vi "HumanExecuteCompitition.vi"(8 "error in (no error)":errorcluster) -> (0 "error out":errorcluster)   [LabVIEW 2023]
doc: "Execute for Human\n\ninput:\n error in (cluster)\n\noutput:\n error out (cluster)"
uses:
  <vilib>/Rock Robotics/WPI/Joystick/XBox Buttons Indexer.ctl
  <vilib>/Rock Robotics/WPI/Joystick/XBox Axes Indexer.ctl
  <vilib>/Rock Robotics/WPI/ThirdParty/JAS_Junk/TrajLib/VI/BoolCmd_Send_Internal.vi
  <vilib>/Rock Robotics/WPI/ThirdParty/JAS_Junk/TrajLib/VI/BoolCmd_ObtainQueue.vi
  HumanGlobal.vi
  <vilib>/Rock Robotics/Network Tables/NT Write String.vi
  <vilib>/Rock Robotics/WPI/ThirdParty/JAS_Junk/TrajLib/Trajectory_Library.lvlib
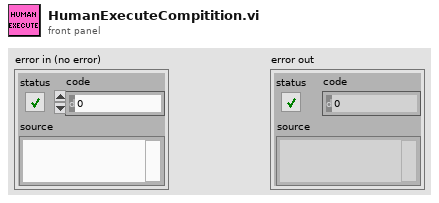
[diagram p1: front panel]
types:
  T1 = typedef "XBox Axes Indexer.ctl" = enum16{"Left X", "Left Y", "Left Trigger", "Right Trigger", "Right X", "Right Y"}
  T2 = typedef "XBox Buttons Indexer.ctl" = enum16{"A", "B", "X", "Y", "Left Bumper", "Right Bumper", "Back", "Start", "Left Joystick", "Right Joystick"}
  T3 = typedef "WPI_JoystickDevRef.ctl" = cluster{"Device":T4}
  T4 = typedef "WPI_JoystickDeviceEnum.ctl" = enum16{"USB 0", "USB 1", "USB 2", "USB 3", "USB 4", "USB 5"}
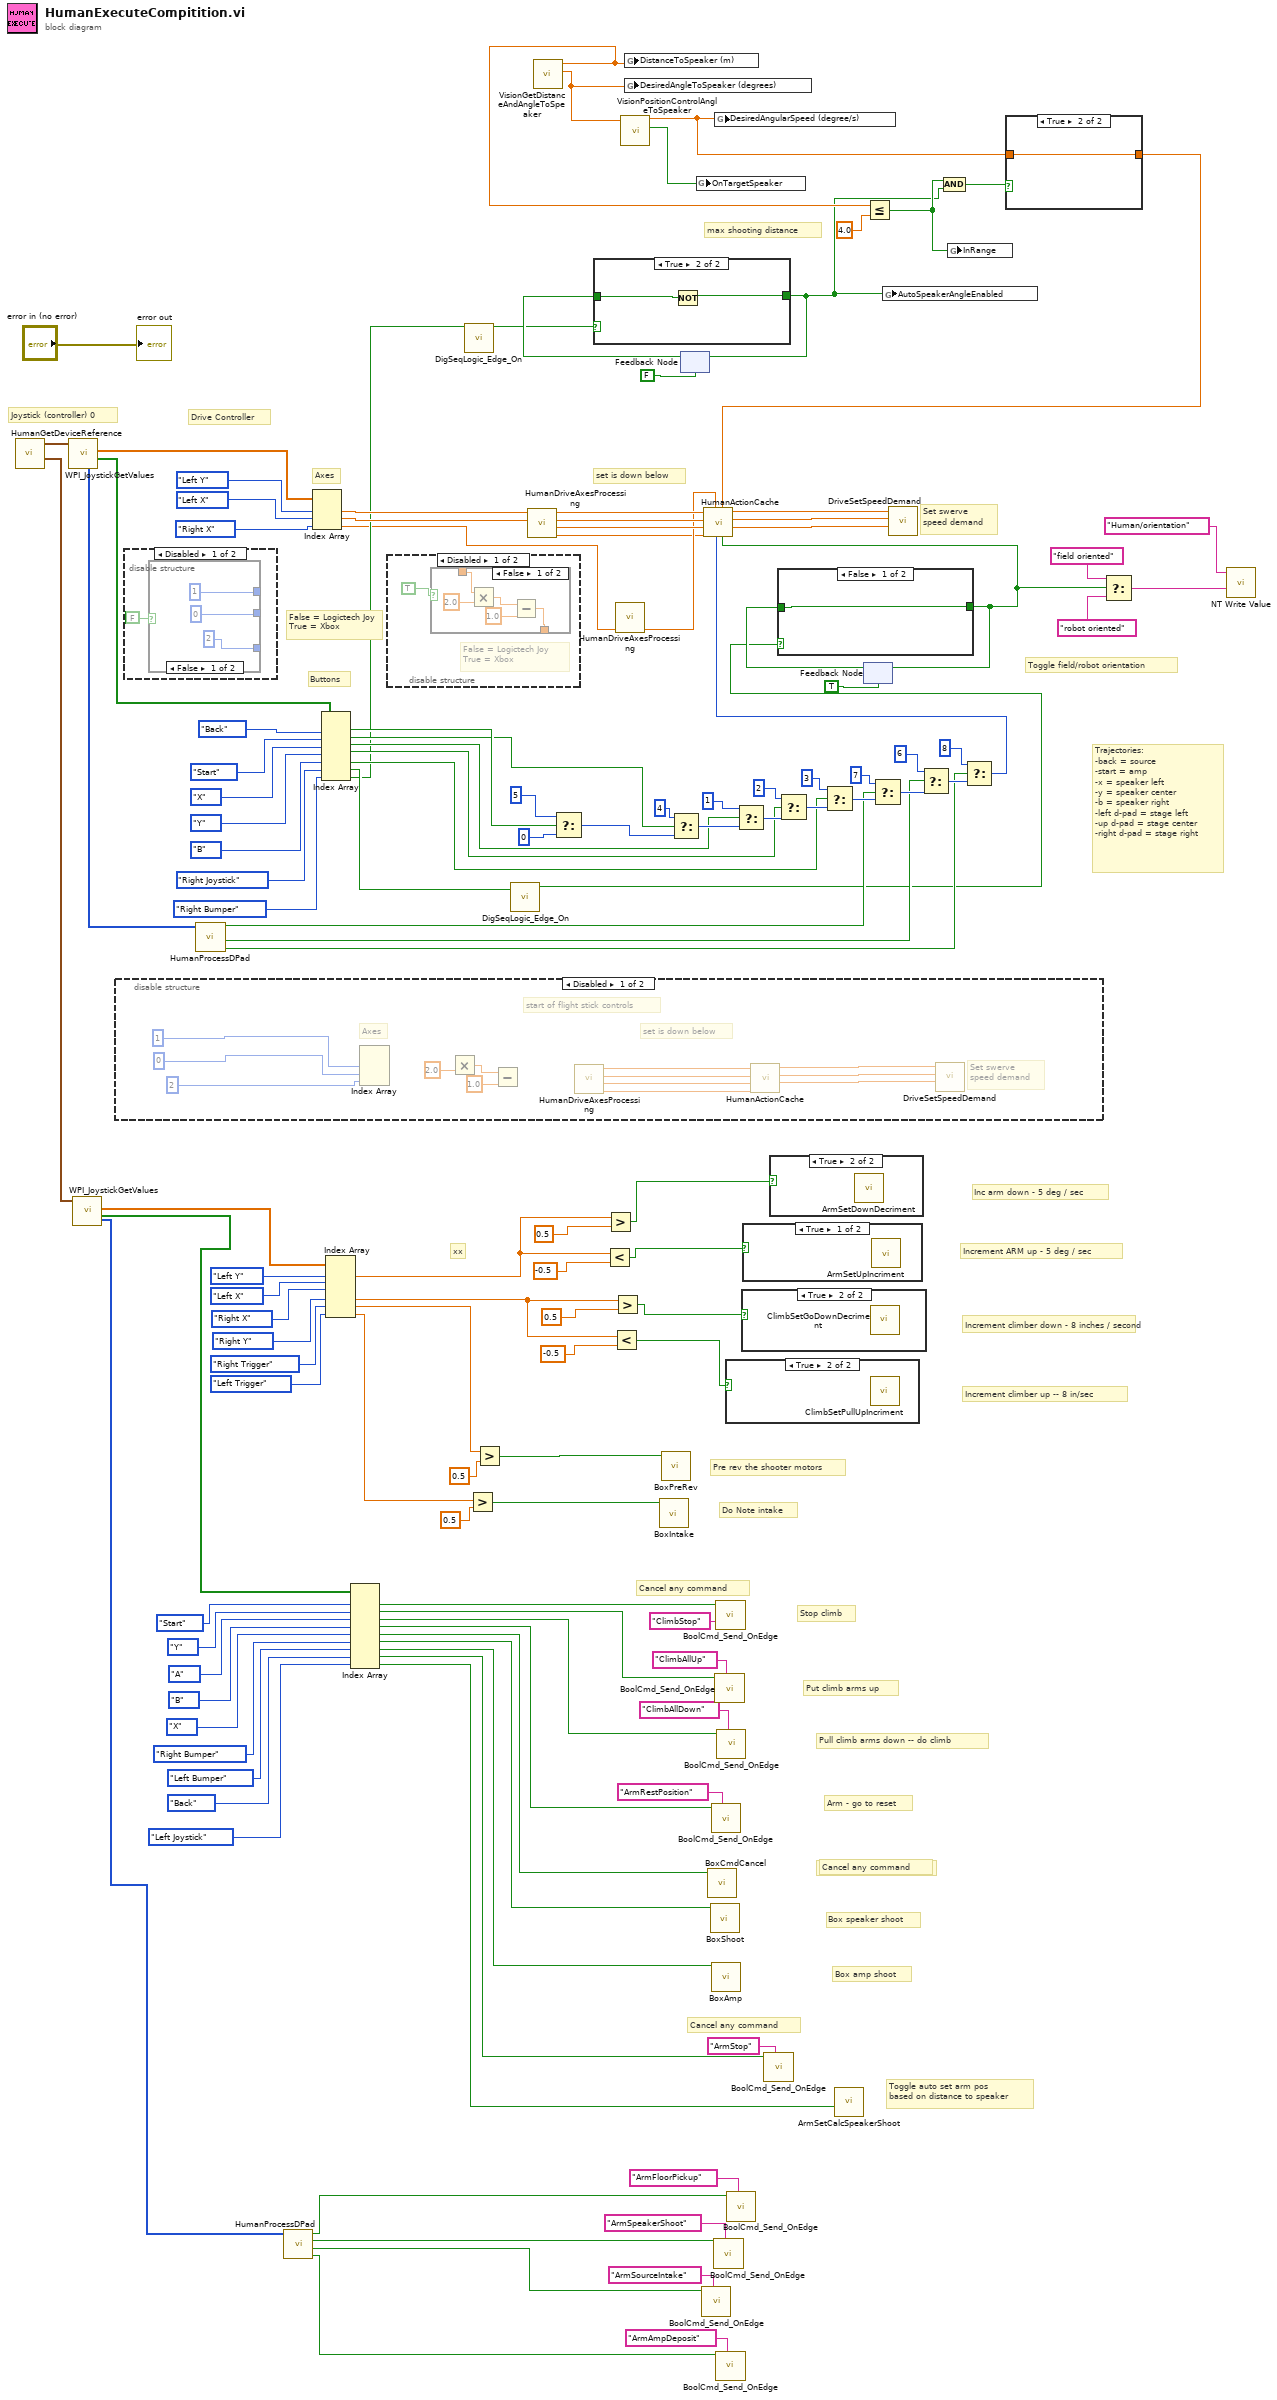
[diagram p0: block diagram]
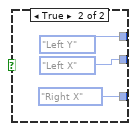
[diagram p3: hidden frame]
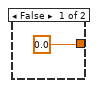
[diagram p8: hidden frame]
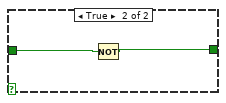
[diagram p9: hidden frame]
diagram:
  # "False = Logictech Joy\nTrue = Xbox"
  # "Toggle auto set arm pos\nbased on distance to speaker"
  # "Box amp shoot"
  # "Box speaker shoot"
  # "Box - cancel any action"
  # "Arm - go to reset"
  # "Pull climb arms down -- do climb"
  # "Put climb arms up"
  # "Stop climb"
  # "Increment ARM up - 5 deg / sec"
  # "Increment climber up -- 8 in/sec"
  # "Do Note intake"
  # "Pre rev the shooter motors"
  # "max shooting distance"
  # "Toggle field/robot orientation"
  # "Increment climber down - 8 inches / second"
  # "xx"
  # "Cancel any command"
  # "Cancel any command"
  # "Inc arm down - 5 deg / sec"
  # "Trajectories:\n-back = source\n-start = amp\n-x = speaker left\n-y = speaker center\n-b = speaker right\n-left d-pad = stage left\n-up d-pad = stage center\n-right d-pad = stage right"
  # "Buttons"
  # "Axes"
  # "Cancel any command"
  # "set is down below"
  # "Set swerve\nspeed demand"
  # "Joystick (controller) 0"
  # "Drive Controller"
  n1 = call "HumanGetDeviceReference.vi"() -> ("Aux Joy"=w116:T3, "Driver Joy"=w120:T3)  [unwired: 9 in, 1 out]
  n2 = call <vilib>:"WPI_JoystickGetValues.vi"("JoystickDevRef"=w120) -> ("Buttons"=w93:bool[], "Axes"=w102:dbl[], "POVs"=w129:i16[])  [unwired: 6 in, 2 out]
  n3 = call <vilib>:"WPI_JoystickGetValues.vi"("JoystickDevRef"=w116) -> ("Buttons"=w106:bool[], "Axes"=w115:dbl[], "POVs"=w68:i16[])  [unwired: 6 in, 2 out]
  n4 = disable-structure shown="Disabled" {
    frame Disabled {
      # "start of flight stick controls"
      # "Axes"
      # "set is down below"
      # "Set swerve\nspeed demand"
      n5 = Index Array(index #1=1, index #2=0, index #3=2) -> ()  [unwired: 1 in, 3 out]
      n6 = Multiply(y=2.0) -> (x*y=w132:dbl)  [unwired: 1 in]
      n7 = Subtract(x=w132, y=1.0) -> ()  [unwired: 1 out]
      n8 = call "HumanDriveAxesProcessing.vi"() -> ("Right X"=w137:dbl, "Right Y"=w142:dbl, "Left X"=w143:dbl, "Left Y"=w141:dbl)  [unwired: 8 in]
      n9 = call "HumanActionCache.vi"("Right X"=w137, "Right Y"=w142, "Left X"=w143, "Left Y"=w141) -> ("AMotorDemand"=w140:dbl, "YMotorDemand"=w139:dbl, "XMotorDemand"=w138:dbl)  [unwired: 5 in]
      n10 = call "DriveSetSpeedDemand.vi"("ASpeedDemand (d/s)"=w140, "YSpeedDemand (ft/s)"=w139, "XSpeedDemand (ft/s)"=w138) -> ()  [unwired: 9 in]
    }
    frame Enabled {
    }
  }
  n11 = disable-structure shown="Disabled" {
    frame Disabled {
      n12 = case shown="False" FALSE {
        tunnel: [1 XBox_Axes_Indexer."Left Y" ("XBox Axes")] -> _
        tunnel: [0 XBox_Axes_Indexer."Left X" ("XBox Axes")] -> _
        tunnel: [2 XBox_Axes_Indexer."Right X" ("XBox Axes")] -> _
        frame False {
        }
        frame True {
        }
      }
    }
    frame Enabled {
    }
  }
  n13 = call "HumanProcessDPad.vi"("POV"=w129) -> ("Right"=w46:bool, "Left"=w47:bool, "Up"=w48:bool)  [unwired: 7 in, 1 out]
  n14 = call "HumanProcessDPad.vi"("POV"=w68) -> ("Right"=w65:bool, "Left"=w63:bool, "Down"=w64:bool, "Up"=w66:bool)  [unwired: 7 in]
  n15 = Index Array(array=w102, index #1=XBox_Axes_Indexer."Left Y" ("XBox Axes"), index #2=XBox_Axes_Indexer."Left X" ("XBox Axes"), index #3=XBox_Axes_Indexer."Right X" ("XBox Axes")) -> (element #1=w128:dbl, element #2=w127:dbl, element #3=w5:dbl)
  n16 = Index Array(array=w93, index #1=XBox_Buttons_Indexer."Back" ("Nothing"), index #2=XBox_Buttons_Indexer."Start" ("Nothing"), index #3=XBox_Buttons_Indexer."X" ("Nothing"), index #4=XBox_Buttons_Indexer."Y" ("Nothing"), index #5=XBox_Buttons_Indexer."B" ("Nothing"), index #6=XBox_Buttons_Indexer."Right Joystick" ("Nothing"), index #7=XBox_Buttons_Indexer."Right Bumper" ("Nothing")) -> (element #1=w62:bool, element #2=w52:bool, element #3=w51:bool, element #4=w50:bool, element #5=w49:bool, element #6=w32:bool, element #7=w12:bool)
  n17 = Index Array(array=w115, index #1=XBox_Axes_Indexer."Left Y" ("XBox Axes"), index #2=XBox_Axes_Indexer."Left X" ("XBox Axes"), index #3=XBox_Axes_Indexer."Right X" ("XBox Axes"), index #4=XBox_Axes_Indexer."Right Y" ("XBox Axes"), index #5=XBox_Axes_Indexer."Right Trigger" ("XBox Axes"), index #6=XBox_Axes_Indexer."Left Trigger" ("XBox Axes")) -> (element #1=w82:dbl, element #4=w74:dbl, element #5=w100:dbl, element #6=w97:dbl)  [unwired: 2 out]
  n18 = Index Array "Index Array"(array=w106, index #1=XBox_Buttons_Indexer."Start" ("Nothing"), index #2=XBox_Buttons_Indexer."Y" ("OpenCloseClaw"), index #3=XBox_Buttons_Indexer."A" ("GrabberIn"), index #4=XBox_Buttons_Indexer."B" ("GrabberOut"), index #5=XBox_Buttons_Indexer."X" ("Nothing"), index #6=XBox_Buttons_Indexer."Right Bumper" ("Nothing"), index #7=XBox_Buttons_Indexer."Left Bumper" ("Nothing"), index #8=XBox_Buttons_Indexer."Back" ("Place Cone"), index #9=XBox_Buttons_Indexer."Left Joystick" ("Place Cone")) -> (element #1=w73:bool, element #2=w72:bool, element #3=w71:bool, element #4=w70:bool, element #5=w94:bool, element #6=w101:bool, element #7=w95:bool, element #8=w69:bool, element #9=w6:bool)
  n19 = disable-structure shown="Disabled" {
    frame Disabled {
      # "False = Logictech Joy\nTrue = Xbox"
      n20 = case shown="False" TRUE {
        tunnel: [w153 w157] -> _
        tunnel: _ -> [w156 w157]
        frame False {
          n21 = Multiply(x=w156, y=2.0) -> (x*y=w154:dbl)
          n22 = Subtract(x=w154, y=1.0) -> (x-y=w153:dbl)
        }
        frame True {
        }
      }
    }
    frame Enabled {
    }
  }
  n23 = call <vilib>:"DigSeqLogic_Edge_On.vi"("Input"=w12) -> ("On Edge"=w13:bool)  [unwired: 10 in]
  n24 = Greater?(x=w97, y=0.5) -> (0:w96:bool)
  n25 = Greater?(x=w100, y=0.5) -> (0:w9:bool)
  n26 = call <vilib>:"DigSeqLogic_Edge_On.vi"("Input"=w32) -> ("On Edge"=w30:bool)  [unwired: 10 in]
  n27 = call "HumanDriveAxesProcessing.vi"("Left X"=w127, "Left Y"=w128) -> ("Right X"=w4:dbl, "Right Y"=w125:dbl, "Left X"=w126:dbl, "Left Y"=w124:dbl)  [unwired: 6 in]
  n28 = call "VisionGetDistanceAndAngleToSpeaker.vi"() -> ("DesiredAngle"=w23:dbl, "Distance"=w21:dbl)  [unwired: 10 in]
  n29 = Select(t=5, s=w62, f=0) -> (s? t:f=w59:i32)
  n30 = Less?(x=w82, y=-0.5) -> (x < y?=w35:bool)
  n31 = Greater?(x=w82, y=0.5) -> (0:w34:bool)
  n32 = Less?(x=w74, y=-0.5) -> (x < y?=w37:bool)
  n33 = Greater?(x=w74, y=0.5) -> (0:w36:bool)
  n34 = call "HumanDriveAxesProcessing.vi"("Right X"=w5) -> ("Right X"=w8:dbl)  [unwired: 7 in, 3 out]
  n35 = call "VisionPositionControlAngleToSpeaker.vi"("TargetAngle"=w23) -> ("OnTargetSpeaker"=w22:bool, "DesiredAngularSpeed (degree/s)"=w19:dbl)  [unwired: 9 in]
  n36 = global write "HumanGlobal.vi" "DistanceToSpeaker (m)"(w21) -> ()
  n37 = global write "HumanGlobal.vi" "DesiredAngleToSpeaker (degrees)"(w23) -> ()
  n38 = call "BoxIntake.vi"("Box intake"=w96) -> ()  [unwired: 10 in, 1 out]
  n39 = call "BoxPreRev.vi"("PreRev"=w9) -> ()  [unwired: 10 in, 1 out]
  n40 = Select(t=4, s=w52, f=w59) -> (s? t:f=w58:i32)
  n41 = feedback #1(FALSE) -> (w15:bool)
  n42 = case shown="True" w13 {
    tunnel: w15 -> [w158 w160]
    tunnel: [w158 w159] -> w11
    frame False {
    }
    frame True {
      n43 = Not(x=w160) -> (.not. x?=w159:bool)
    }
  }
  n44 = feedback-in #1(w11) -> ()
  n45 = global write "HumanGlobal.vi" "OnTargetSpeaker"(w22) -> ()
  n46 = call <vilib>:"BoolCmd_Send_OnEdge.vi"("Command Name"="ArmSourceIntake", "Value"=w63) -> ()  [unwired: 9 in, 1 out]
  n47 = call "BoxCmdCancel.vi"("box cancel"=w94) -> ()  [unwired: 11 in]
  n48 = call "BoxShoot.vi"("Box shoot"=w101) -> ()  [unwired: 10 in, 1 out]
  n49 = call <vilib>:"BoolCmd_Send_OnEdge.vi"("Command Name"="ArmRestPosition", "Value"=w70) -> ()  [unwired: 9 in, 1 out]
  n50 = call "BoxAmp.vi"("box amp"=w95) -> ()  [unwired: 11 in]
  n51 = call <vilib>:"BoolCmd_Send_OnEdge.vi"("Command Name"="ArmSpeakerShoot", "Value"=w64) -> ()  [unwired: 9 in, 1 out]
  n52 = global write "HumanGlobal.vi" "DesiredAngularSpeed (degree/s)"(w19) -> ()
  n53 = call <vilib>:"BoolCmd_Send_OnEdge.vi"("Command Name"="ClimbAllUp", "Value"=w72) -> ()  [unwired: 9 in, 1 out]
  n54 = call <vilib>:"BoolCmd_Send_OnEdge.vi"("Command Name"="ClimbStop", "Value"=w73) -> ()  [unwired: 9 in, 1 out]
  n55 = call <vilib>:"BoolCmd_Send_OnEdge.vi"("Command Name"="ArmAmpDeposit", "Value"=w65) -> ()  [unwired: 9 in, 1 out]
  n56 = call <vilib>:"BoolCmd_Send_OnEdge.vi"("Command Name"="ClimbAllDown", "Value"=w71) -> ()  [unwired: 9 in, 1 out]
  n57 = case shown="True" w37 {
    frame False {
    }
    frame True {
      n58 = call "ClimbSetPullUpIncriment.vi"() -> ()  [unwired: 11 in, 1 out]
    }
  }
  n59 = call <vilib>:"BoolCmd_Send_OnEdge.vi"("Command Name"="ArmFloorPickup", "Value"=w66) -> ()  [unwired: 9 in, 1 out]
  n60 = Select(t=1, s=w51, f=w58) -> (s? t:f=w57:i32)
  n61 = case shown="True" w36 {
    frame False {
    }
    frame True {
      n62 = call "ClimbSetGoDownDecriment.vi"() -> ()  [unwired: 11 in, 1 out]
    }
  }
  n63 = case shown="True" w35 {
    frame True {
      n64 = call "ArmSetUpIncriment.vi"() -> ()  [unwired: 11 in, 1 out]
    }
    frame False {
    }
  }
  n65 = call <vilib>:"BoolCmd_Send_OnEdge.vi"("Command Name"="ArmStop", "Value"=w69) -> ()  [unwired: 9 in, 1 out]
  n66 = case shown="True" w34 {
    frame False {
    }
    frame True {
      n67 = call "ArmSetDownDecriment.vi"() -> ()  [unwired: 11 in, 1 out]
    }
  }
  n68 = Select(t=2, s=w50, f=w57) -> (s? t:f=w56:i32)
  n69 = Select(t=3, s=w49, f=w56) -> (s? t:f=w55:i32)
  n70 = call "ArmSetCalcSpeakerShoot.vi"("ArmCalcSpeaker"=w6) -> ()  [unwired: 10 in, 1 out]
  n71 = feedback #2(TRUE) -> (w31:bool)
  n72 = case shown="False" w30 {
    tunnel: w31 -> [w161 w163]
    tunnel: [w161 w162] -> w28
    frame False {
    }
    frame True {
      n73 = Not(x=w163) -> (.not. x?=w162:bool)
    }
  }
  n74 = feedback-in #2(w28) -> ()
  n75 = Less Or Equal?(x=w21, y=4.0) -> (x <= y?=w18:bool)
  n76 = Select(t=7, s=w48, f=w55) -> (s? t:f=w54:i32)
  n77 = global write "HumanGlobal.vi" "AutoSpeakerAngleEnabled"(w11) -> ()
  n78 = Select(t=6, s=w47, f=w54) -> (s? t:f=w53:i32)
  n79 = And(x=w18, y=w11) -> (x .and. y?=w17:bool)
  n80 = global write "HumanGlobal.vi" "InRange"(w18) -> ()
  n81 = Select(t=8, s=w46, f=w53) -> (s? t:f=w38:i32)
  n82 = case shown="True" w17 {
    tunnel: w19 -> [_ w165]
    tunnel: [0.0 w165] -> w10
    frame False {
    }
    frame True {
    }
  }
  n83 = call "HumanActionCache.vi"("Enable Field Oriented Drive"=w28, "AutoSpeakerAngle"=w10, "State"=w38, "Rotation"=w8, "Right X"=w4, "Right Y"=w125, "Left X"=w126, "Left Y"=w124) -> ("AMotorDemand"=w123:dbl, "YMotorDemand"=w122:dbl, "XMotorDemand"=w121:dbl)  [unwired: 1 in]
  n84 = call "DriveSetSpeedDemand.vi"("ASpeedDemand (d/s)"=w123, "YSpeedDemand (ft/s)"=w122, "XSpeedDemand (ft/s)"=w121) -> ()  [unwired: 9 in]
  n85 = Select(t="field oriented", s=w28, f="robot oriented") -> (s? t:f=w25:string)
  n86 = call-poly <vilib>:"NT Write Value.vi"("value"=w25, "name"="Human/orientation") -> ()  [unwired: 9 in, 1 out]
  "error out" <- "error in (no error)"
